vi "Replace Actual Class Objects on Front Panel with Test Class.vi"(8 "error in (no error)":errorcluster, 11 "Test Double Factory in":refnum<class "Test Double Factory.lvclass">) -> (0 "error out":errorcluster, 3 "Test Double Factory out":refnum<class "Test Double Factory.lvclass">)   [LabVIEW 2020, in "Test Double Factory.lvclass"]
uses:
  Test Double Factory.lvclass
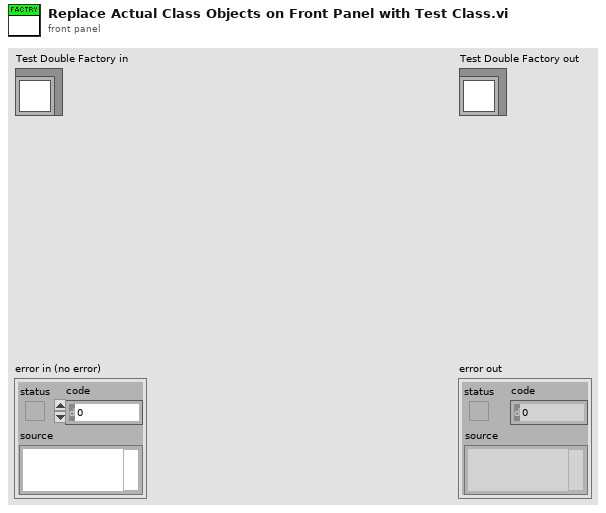
[diagram p1: front panel]
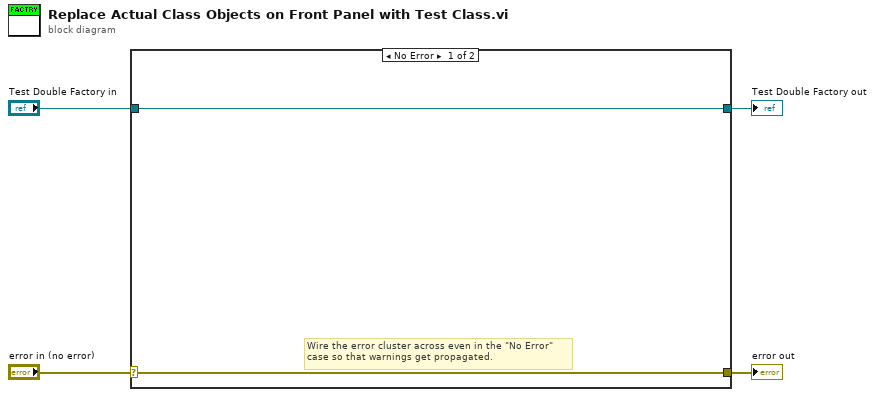
[diagram p0: block diagram]
diagram:
  n1 = case shown="No Error" "error in (no error)" {
    selector: "error in (no error)" -> [w5 w8]
    tunnel: [w5 w8] -> w3
    tunnel: [w6 w7] -> w1
    tunnel: "Test Double Factory in" -> [w6 w7]
    frame No Error {
      # "Wire the error cluster across even in the \"No Error\"\ncase so that warnings get propagated."
    }
    frame Error {
    }
  }
  "error out" <- w3
  "Test Double Factory out" <- w1
